vi "Is_TopLevel.vi"(8 "error in (no error)":errorcluster, 11 "AB_Source_VI in":refnum<class "AB_Source_VI.lvclass">) -> (0 "error out":errorcluster, 1 "openVIreference":bool, 2 "path":path, 3 "AB_Source_VI out":refnum<class "AB_Source_VI.lvclass">, 5 "readLinker":bool)   [LabVIEW 2020, in "AB_Source_VI.lvclass"]
uses:
  <vilib>/AppBuilder/AB_Classes/Source/VI/AB_Source_VI.lvclass
  e:/builds/penguin/labview/branches/2020/dev/dist/vi.lib/AppBuilder/AB_Classes/Source/AB_Source.lvclass
  <vilib>/AppBuilder/AB_Classes/Source/VI/AB_Source_VI.lvclass/AB_Source_VI.ctl
  <vilib>/AppBuilder/AB_Classes/Source/AB_Source.lvclass
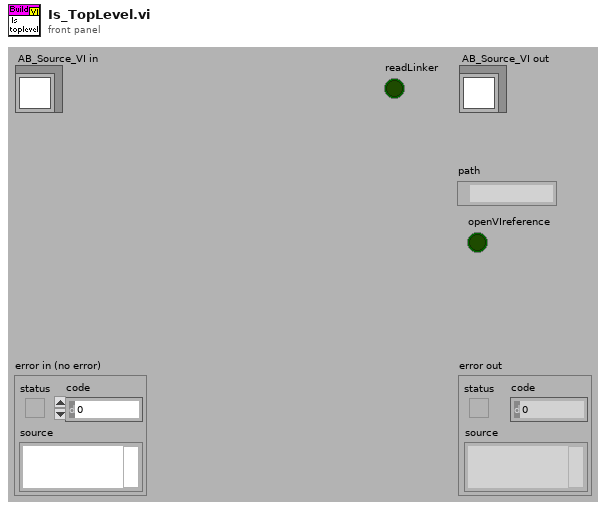
[diagram p1: front panel]
types:
  T1 = typedef "AB_Source.ctl" = cluster{"path":path, "itemID":string, "parentIndex":i32, "sourceInclusion":T2, "destinationIndex":i32, "properties":T3[], "newName":string, "lvfile":bool, "valid":bool, "eng_inBuild":bool, "eng_isNonVILink":bool, "Amalgamation":bool, "Amalgamation Piece":bool, "eng_delimitedName":string, "preventRename":bool}
  T2 = typedef "AB_Source_Inclusion.ctl" = enum16{"IncludeIfReferenced", "Include", "Exclude", "TopLevel"}
  T3 = typedef "AB_Source_Properties.ctl" = cluster{"sourcePropertyType":T4, "value":variant}
  T4 = typedef "AB_Source_Property_Type.ctl" = enum16{"Remove block diagram", "Remove front panel", "Password", "Window has title bar", "Show menu bar", "Show vertical scroll bar", "Show horizontal scroll bar", "Show toolbar", "Show Abort button", "Show fp when called", "Window behavior", "Allow user to close window", "Window run-time position", "Run when opened", "Allow debugging", "Auto error handling", "Generate guard code", "Use stack variables", "Expression folding", "Integer only", "Inline subVI"}
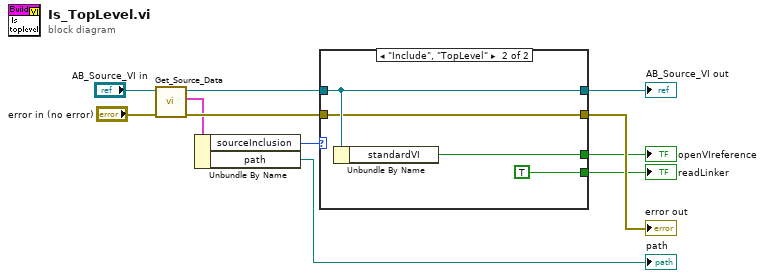
[diagram p0: block diagram]
diagram:
  n1 = call <vilib>:"Get_Source_Data.vi"("error in (no error)"="error in (no error)", "Class in"="AB_Source_VI in") -> ("error out"=w6:errorcluster, "data"=w5:T1, "Class out"=w8:refnum<class "AB_Source_VI.lvclass">)  [unwired: 7 in]
  n2 = Unbundle By Name(w5) -> ("sourceInclusion"=w4:T2, "path"=→"path":path)
  n3 = case shown="\"Include\", \"TopLevel\"" w4 {
    tunnel: w8 -> [w13 w16]
    tunnel: w6 -> [w12 w15]
    tunnel: [w13 w16] -> w11
    tunnel: [w12 w15] -> w10
    tunnel: [_ w17] -> w1
    tunnel: [_ TRUE] -> w2
    frame Default {
    }
    frame "Include", "TopLevel" {
      n4 = Unbundle By Name(w16) -> ("standardVI"=w17:bool)
    }
  }
  "error out" <- w10
  "openVIreference" <- w1
  "AB_Source_VI out" <- w11
  "readLinker" <- w2
